vi "Interfata.vi"() -> ()   [LabVIEW 2024]
panel:
  out "standard error":string
  out "Application Directory":path
  out "standard output":string
  out "resulting string":string
  out "Acuratete":string
  out "Instrument identificat 2":string
  in  "Classify":bool
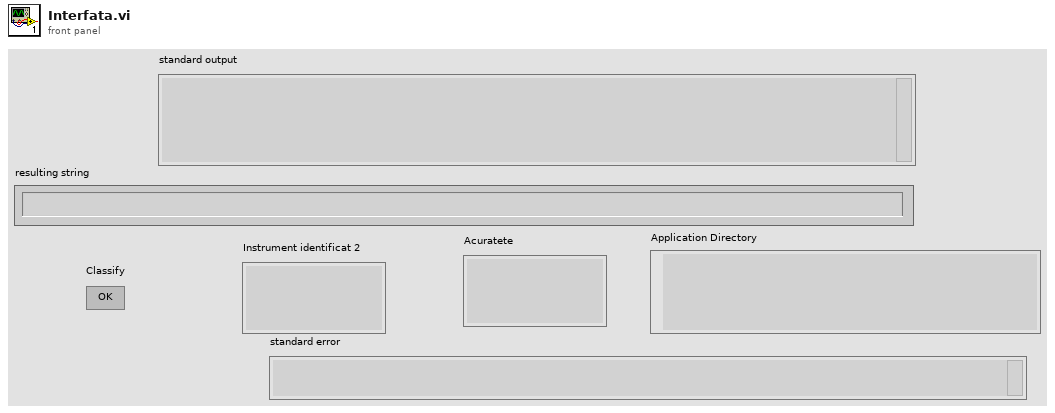
[diagram p1: front panel]
types:
  T1 = cluster{"instrument":string, "confidence":string}
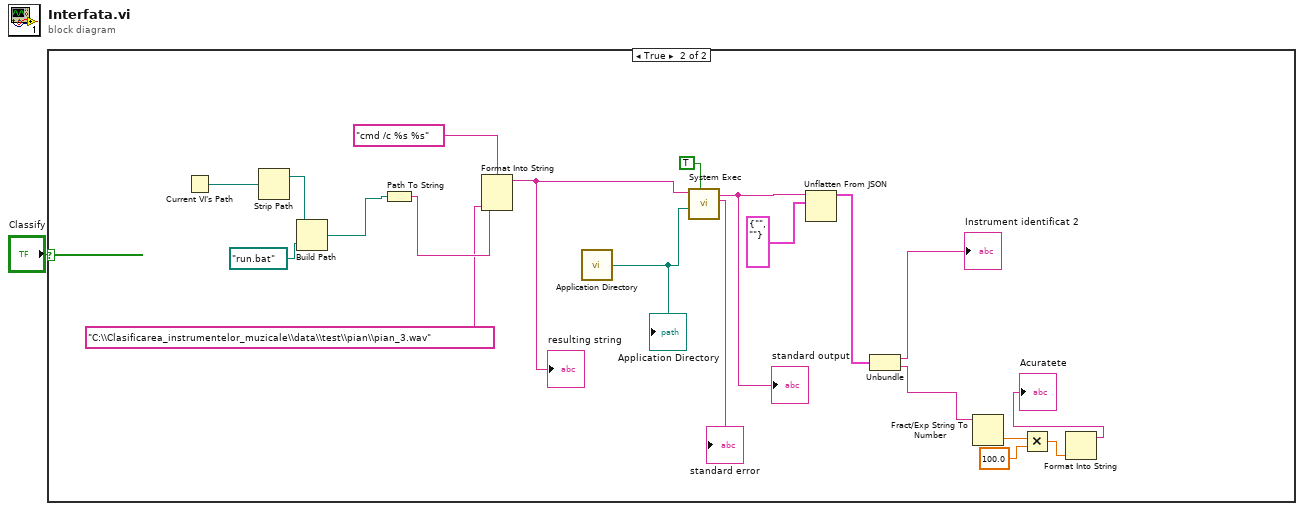
[diagram p0: block diagram]
diagram:
  n1 = case shown="True" "Classify" {
    frame False {
    }
    frame True {
      n2 = Current VI's Path() -> (path=w13:path)
      n3 = Strip Path(path=w13) -> (stripped path=w12:path)  [unwired: 1 out]
      n4 = Build Path(base path=w12, name or relative path=path "run.bat") -> (appended path=w11:path)
      n5 = Path To String(path=w11) -> (string=w10:string)
      n6 = Format Into String "Format Into String"(format string="cmd /c %s %s", w10, "C:\\Clasificarea_instrumentelor_muzicale\\data\\test\\pian\\pian_3.wav") -> (resulting string=w21:string)  [unwired: 2 in, 1 out]
      "resulting string" <- w21
      n7 = call <vilib>:"Application Directory.vi"() -> ("Application Directory"=w14:path)
      "Application Directory" <- w14
      n8 = call <vilib>:"System Exec.vi"("wait until completion? (T)"=TRUE, "working directory"=w14, "command line"=w21) -> ("standard error"=→"standard error":string, "standard output"=w15:string)  [unwired: 5 in, 2 out]
      "standard output" <- w15
      n9 = Unflatten From JSON(JSON string=w15, type and defaults=T1 {"instrument"="", "confidence"=""} ("Cluster")) -> (value=w19:T1)  [unwired: 5 in, 1 out]
      n10 = Unbundle(w19) -> ("instrument"=→"Instrument identificat 2":string, "confidence"=w16:string)
      n11 = Fract/Exp String To Number(string=w16) -> (number=w18:dbl)  [unwired: 3 in, 1 out]
      n12 = Multiply(x=w18, y=100.0) -> (x*y=w17:dbl)
      n13 = Format Into String(w17) -> (resulting string=→"Acuratete":string)  [unwired: 3 in, 1 out]
    }
  }
